vi "Continued Fraction.vi"(2 "B":dbl[](array[numeric]) format="%.2f", 3 "A":dbl[](array[numeric]) format="%.2f") -> (0 "error":i32 format="%.2f", 1 "result":dbl format="%.2f")   [LabVIEW 2010, in "NI_Gmath.lvlib"]
doc: "Evaluates the continued fraction of two sequences (a[0], a[1], ..., a[n]) and (b[0], b[1], ..., b[n])."
uses:
  NI_Gmath.lvlib
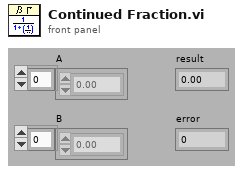
[diagram p1: front panel]
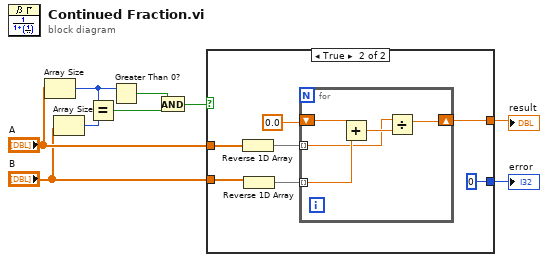
[diagram p0: block diagram]
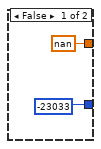
[diagram p2: hidden frame]
diagram:
  n1 = Array Size(array="A") -> (size(s)=w4:i32)
  n2 = Array Size(array="B") -> (size(s)=w5:i32)
  n3 = Equal?(x=w4, y=w5) -> (x = y?=w2:bool)
  n4 = Greater Than 0?(x=w4) -> (x > 0?=w3:bool)
  n5 = And(x=w3, y=w2) -> (x .and. y?=w1:bool)
  n6 = case shown="True" w1 {
    tunnel: [nan w18] -> w9
    tunnel: "B" -> [_ w15]
    tunnel: "A" -> [_ w14]
    tunnel: [-23033 0] -> w8
    frame False {
    }
    frame True {
      n7 = Reverse 1D Array(array=w14) -> (reversed array=w17:dbl[])
      n8 = Reverse 1D Array(array=w15) -> (reversed array=w16:dbl[])
      n9 = for {
        shift-right: [w20] -> w18
        shift-left: 0.0 -> [w23]
        tunnel: w16 -> [w22] mode=indexing
        tunnel: w17 -> [w19] mode=indexing
        n10 = Add(x=w23, y=w22) -> (x+y=w21:dbl)
        n11 = Divide(x=w19, y=w21) -> (x/y=w20:dbl)
      }
    }
  }
  "result" <- w9
  "error" <- w8
